vi "Execute.vi"(0 "connection ID in":refnum<k5>, 7 "Query":string, 9 "Timeout (60s)":dbl=60.0, 11 "error in (no error)":errorcluster) -> (4 "connection ID out":refnum<k5>, 6 "Data Found?":bool, 8 "Field Names":string[](array[string]), 10 "Recordset data out":string[][](array[string]), 14 "Packet Metadata":T1 {"Server Status" format="%.0x"}, 15 "error out":errorcluster)   [LabVIEW 2014, in "hse-db.lvlib" / "MySQL (TCP).lvlib"]
uses:
  MySQL (TCP).lvlib
  Controls/OK Packet Metadata.ctl
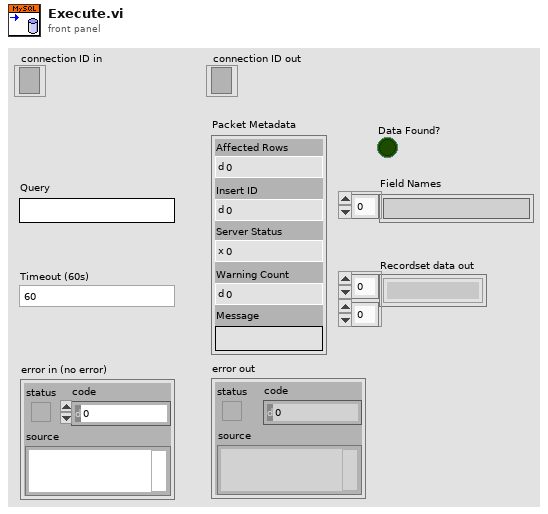
[diagram p1: front panel]
types:
  T1 = typedef "hse-db.lvlib/MySQL (TCP).lvlib/OK Packet Metadata.ctl" = cluster{"Affected Rows":u64, "Insert ID":u64, "Server Status":u16, "Warning Count":u16, "Message":string}
  T2 = typedef "Semaphore RefNum" = refnum<k1>
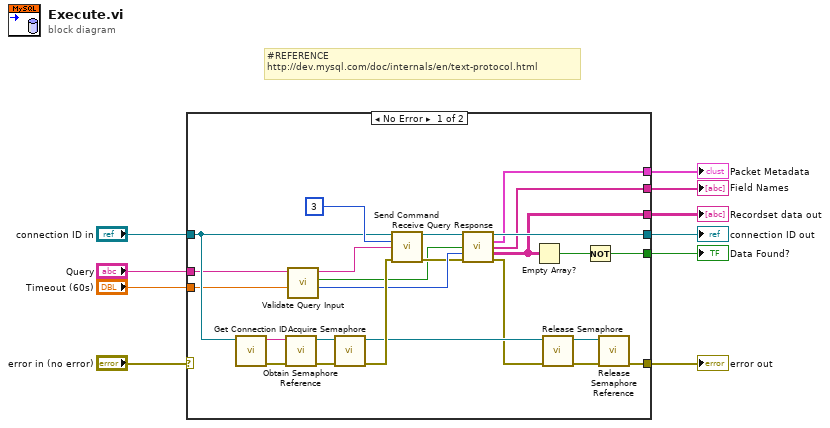
[diagram p0: block diagram]
diagram:
  # "#REFERENCE\nhttp://dev.mysql.com/doc/internals/en/text-protocol.html"
  n1 = case shown="No Error" "error in (no error)" {
    selector: "error in (no error)" -> [_ w37]
    tunnel: [w26 w37] -> w9
    tunnel: [w19 w36] -> w8
    tunnel: "connection ID in" -> [w32 w36]
    tunnel: "Query" -> [w14 _]
    tunnel: "Timeout (60s)" -> [w25 _]
    tunnel: [w18 _] -> w4
    tunnel: [w16 _] -> w3
    tunnel: [w23 _] -> w2
    tunnel: [w17 _] -> w1
    frame No Error {
      n2 = call "Get Connection ID.vi"("TCP Network Connection in"=w32) -> ("Error Out"=w11:errorcluster, "ConnectionID"=w34:string)  [unwired: 9 in]
      n3 = call <vilib>:"Obtain Semaphore Reference.vi"("error in (no error)"=w11, "name (unnamed)"=w34) -> ("error out"=w31:errorcluster, "semaphore"=w33:T2)  [unwired: 3 in, 1 out]
      n4 = call "Validate Query Input.vi"("Timeout (s)"=w25, "Query in"=w14) -> ("Timeout (ms)"=w21:i32, "Call Procedure?"=w12:bool, "Query out"=w13:string)  [unwired: 7 in]
      n5 = call <vilib>:"Acquire Semaphore.vi"("error in (no error)"=w31, "semaphore"=w33) -> ("error out"=w30:errorcluster, "semaphore out"=w29:T2)  [unwired: 3 in, 1 out]
      n6 = call "Send Command.vi"("connection ID"=w32, "Command"=u8 3, "Message"=w13, "error in (no error)"=w30) -> ("connection ID out"=w22:refnum<k5>, "error out"=w20:errorcluster)  [unwired: 10 in]
      n7 = call "Receive Query Response.vi"("connection ID"=w22, "Call Procedure?"=w12, "Timeout (60000ms)"=w21, "error in (no error)"=w20) -> ("connection ID out"=w19:refnum<k5>, "OK Packet Metadata"=w18:T1, "Field Names"=w17:string[], "Return Data"=w16:string[][], "error out"=w15:errorcluster)  [unwired: 7 in]
      n8 = Empty Array?(array=w16) -> (empty?=w24:bool)
      n9 = call <vilib>:"Release Semaphore.vi"("error in (no error)"=w15, "semaphore"=w29) -> ("error out"=w27:errorcluster, "semaphore out"=w28:T2)  [unwired: 4 in]
      n10 = Not(x=w24) -> (.not. x?=w23:bool)
      n11 = call <vilib>:"Release Semaphore Reference.vi"("error in (no error)"=w27, "semaphore"=w28) -> ("error out"=w26:errorcluster)  [unwired: 8 in, 1 out]
    }
    frame Error {
    }
  }
  "error out" <- w9
  "connection ID out" <- w8
  "Packet Metadata" <- w4
  "Recordset data out" <- w3
  "Data Found?" <- w2
  "Field Names" <- w1
